vi "Specified version not found--error.vi"(10 "Architecture":T1, 11 "Version":string) -> (0 "error out":errorcluster)   [LabVIEW 2025]
doc: "Indicates that the specified TestStand version was not found."
uses:
  Type Definitions/Architecture--enum.ctl
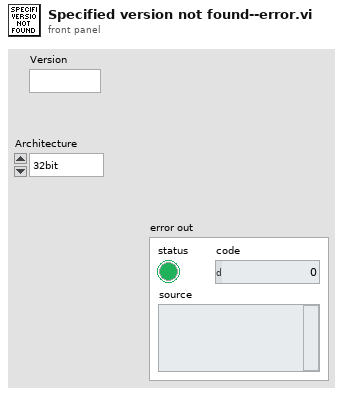
[diagram p1: front panel]
types:
  T1 = typedef "Architecture--enum.ctl" = enum16{"32bit", "64bit"}
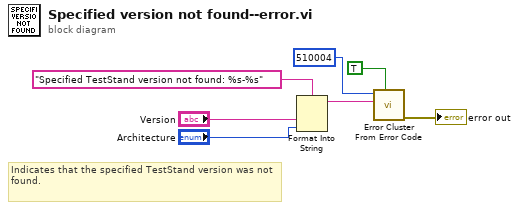
[diagram p0: block diagram]
diagram:
  # "Indicates that the specified TestStand version was not found."
  n1 = Format Into String(format string="Specified TestStand version not found: %s-%s" ("error message (\"\")"), "Version", "Architecture") -> (resulting string=w1:string)  [unwired: 2 in, 1 out]
  n2 = call <vilib>:"Error Cluster From Error Code.vi"("show call chain? (False)"=TRUE, "error message (\"\")"=w1, "error code (0)"=510004) -> ("error out"=→"error out":errorcluster)  [unwired: 6 in]
